vi "Auto Match.vi"() -> ()   [LabVIEW 2018]
panel:
  out "Number Of Iterations":i32
  out "Current Number":u32 format="%#.0f"
  in  "Number To Match":u32=50 max=1000 step=1
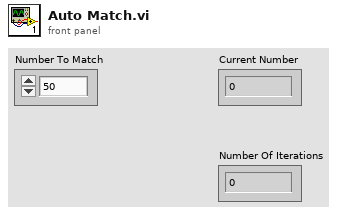
[diagram p1: front panel]
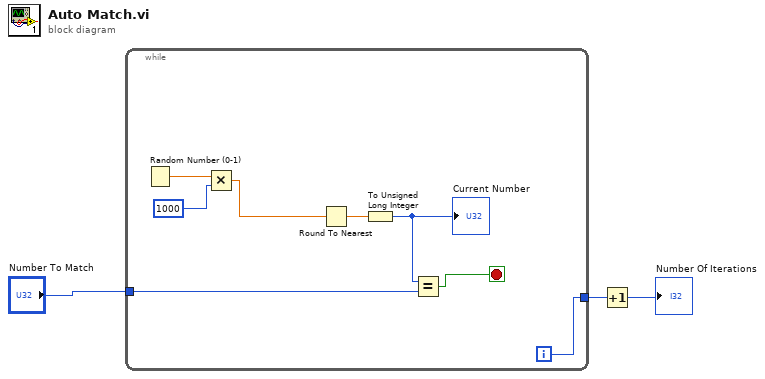
[diagram p0: block diagram]
diagram:
  n1 = while {
    tunnel: "Number To Match" -> [w7]
    tunnel: [w4] -> w1
    i -> [w4]
    stop <- w5 stop-if-true
    n2 = Random Number (0-1)() -> (number: 0 to 1=w11:dbl)
    n3 = Multiply(x=w11, y=1000) -> (x*y=w9:dbl)
    n4 = Round To Nearest(number=w9) -> (nearest integer value=w8:dbl)
    n5 = To Unsigned Long Integer(number=w8) -> (unsigned 32bit integer=w6:u32)
    "Current Number" <- w6
    n6 = Equal?(x=w6, y=w7) -> (x = y?=w5:bool)
  }
  n7 = Increment(x=w1) -> (x+1=→"Number Of Iterations":i32)
